vi "SaveTempData2.vi"(2 "temp data":dbl[][][](array[numeric]), 3 "Exp_params":T3={"filename"="201612011532", "ExpFilePath"=path "\\\\10.0.0.7\\takada2/DATA/HBT6/data/Test/201612011532.h5", "File Ref list"=[16777216, 33554432], "sweep_dim"=[4, 2], "sweep_list"=[], "readout_list"=["ADC0", "ADC1"], "Sweep instrument bools"=[[0, 0], [0, 0], [0, 0], [0, 0], [0, 0], [0, 0], [0, 0], [0, 0], [0, 0], [0, 0], [0, 0], [0, 0], [0, 0], [0, 0], [0, 0], [0, 0], [0, 0], [0, 0], [0, 0], [0, 0], [0, 0], [0, 0], [0, 0], [0, 0], [0, 0], [0, 0], [0, 0], [0, 0], [0, 0], [0, 0], [0, 0]], "Read out instrument bools"=[[1, 0]], "Experimental bool list"=[FALSE, TRUE], "Initial move"=[{"Name"="None", "kind"=100, "Value"=0.0}], "FPGA Ref"=refnum, "Inst_parameters"={"ConfigFilePath"=path "\\\\10.0.0.7\\takada2/DATA/HBT6/data/Configs/HBT6_ramp_1.h5", "Inst_list"=["ADC", "AWG", "Freq", "Power", "sus", "rus", "rls", "sls", "suq", "suu", "sur", "suc", "sul", "ruq", "ruu", "rur", "ruc", "rul", "rlq", "rlu", "rlr", "rlc", "rll", "slq", "slu", "slr", "slc", "sll", "tu", "t", "tl", "fast_sequence"], "fast_mode"=[1, 1], "Wait_times"=[1, 1, 1, 1], "Inst_array"=[{"Kind"=0, "Strings"=["ADC", "", "V", "ADC0;ADC1", "V;V", "1.0;1.0"], "uint64s"=[10, 2, 250000, 0, 100, 10106, 1000000, 1, 0, 1], "Doubles"=[1.0], "DAQmx take out list"=[]}, {"Kind"=7, "Strings"=["AWG", "10.0.0.4", "", "C:\\Documents and Settings\\Bauerle\\Mes documents\\Bautze\\FPGA-clean_works_1.13.6_batchtest\\Python\\AWG", "dummy", "SAWnstrig_v4.py"], "uint64s"=[2, 0, 0, 3, 0, 0, 0, 0, 0, 0, 0, 0, 0, 0], "Doubles"=[1200000000.0, 1.0, 0.0, 1.0, 0.0, 1.0, 0.0, 1.0, 0.0, 1.0, 0.0, 1.0, 0.0], "DAQmx take out list"=[]}, {"Kind"=6, "Strings"=["Freq", "0:19", "GHz"], "uint64s"=[1, 0, 0, 0, 2, 0, 0, 0], "Doubles"=[2.0, -30.0, 200.0, 100.0, 0.0, 6.000999927520752, 9.000000318337698e-06, 30.0, -145.0], "DAQmx take out list"=[]}, {"Kind"=6, "Strings"=["Power", "0:19", "GHz"], "uint64s"=[1, 0, 1, 0, 2, 0, 0, 0], "Doubles"=[2.0, -30.0, 200.0, 100.0, 0.0, 6.000999927520752, 9.000000318337698e-06, 30.0, -145.0], "DAQmx take out list"=[]}, {"Kind"=4, "Strings"=["sus", "10.0.0.2", "mV"], "uint64s"=[0, 1], "Doubles"=[1.0, -1.0, 1.0, -1.0, 1.0], "DAQmx take out list"=[]}, {"Kind"=4, "Strings"=["rus", "10.0.0.2", "mV"], "uint64s"=[0, 2], "Doubles"=[1.0, -1.0, 1.0, -1.0, 1.0], "DAQmx take out list"=[]}, {"Kind"=4, "Strings"=["rls", "10.0.0.2", "mV"], "uint64s"=[0, 3], "Doubles"=[1.0, -1.0, 1.0, -1.0, 1.0], "DAQmx take out list"=[]}, {"Kind"=4, "Strings"=["sls", "10.0.0.2", "mV"], "uint64s"=[0, 4], "Doubles"=[1.0, -1.0, 1.0, -1.0, 1.0], "DAQmx take out list"=[]}, {"Kind"=4, "Strings"=["suq", "10.0.0.2", "V"], "uint64s"=[0, 5], "Doubles"=[0.30000001192092896, -2.0, 1.0, -1.0, 1.0], "DAQmx take out list"=[]}, {"Kind"=4, "Strings"=["suu", "10.0.0.2", "V"], "uint64s"=[0, 6], "Doubles"=[0.30000001192092896, -2.0, 1.0, -1.0, 1.0], "DAQmx take out list"=[]}, {"Kind"=4, "Strings"=["sur", "10.0.0.2", "V"], "uint64s"=[0, 7], "Doubles"=[0.30000001192092896, -2.0, 1.0, -1.0, 1.0], "DAQmx take out list"=[]}, {"Kind"=4, "Strings"=["suc", "10.0.0.2", "V"], "uint64s"=[1, 0], "Doubles"=[0.30000001192092896, -2.0, 1.0, -1.0, 1.0], "DAQmx take out list"=[]}, {"Kind"=4, "Strings"=["sul", "10.0.0.2", "V"], "uint64s"=[1, 1], "Doubles"=[0.30000001192092896, -2.0, 1.0, -1.0, 1.0], "DAQmx take out list"=[]}, {"Kind"=4, "Strings"=["ruq", "10.0.0.2", "V"], "uint64s"=[1, 2], "Doubles"=[0.30000001192092896, -2.0, 1.0, -1.0, 1.0], "DAQmx take out list"=[]}, {"Kind"=4, "Strings"=["ruu", "10.0.0.2", "V"], "uint64s"=[1, 3], "Doubles"=[0.30000001192092896, -2.0, 1.0, -1.0, 1.0], "DAQmx take out list"=[]}, {"Kind"=4, "Strings"=["rur", "10.0.0.2", "V"], "uint64s"=[1, 5], "Doubles"=[0.30000001192092896, -2.0, 1.0, -1.0, 1.0], "DAQmx take out list"=[]}, {"Kind"=4, "Strings"=["ruc", "10.0.0.2", "V"], "uint64s"=[1, 6], "Doubles"=[0.30000001192092896, -2.0, 1.0, -1.0, 1.0], "DAQmx take out list"=[]}, {"Kind"=4, "Strings"=["rul", "10.0.0.2", "V"], "uint64s"=[1, 7], "Doubles"=[0.30000001192092896, -2.0, 1.0, -1.0, 1.0], "DAQmx take out list"=[]}, {"Kind"=4, "Strings"=["rlq", "10.0.0.2", "V"], "uint64s"=[2, 0], "Doubles"=[0.30000001192092896, -2.0, 1.0, -1.0, 1.0], "DAQmx take out list"=[]}, {"Kind"=4, "Strings"=["rlu", "10.0.0.2", "V"], "uint64s"=[2, 1], "Doubles"=[0.30000001192092896, -2.0, 1.0, -1.0, 1.0], "DAQmx take out list"=[]}, {"Kind"=4, "Strings"=["rlr", "10.0.0.2", "V"], "uint64s"=[2, 2], "Doubles"=[0.30000001192092896, -2.0, 1.0, -1.0, 1.0], "DAQmx take out list"=[]}, {"Kind"=4, "Strings"=["rlc", "10.0.0.2", "V"], "uint64s"=[2, 3], "Doubles"=[0.30000001192092896, -2.0, 1.0, -1.0, 1.0], "DAQmx take out list"=[]}, {"Kind"=4, "Strings"=["rll", "10.0.0.2", "V"], "uint64s"=[2, 4], "Doubles"=[0.30000001192092896, -2.0, 1.0, -1.0, 1.0], "DAQmx take out list"=[]}, {"Kind"=4, "Strings"=["slq", "10.0.0.2", "V"], "uint64s"=[2, 5], "Doubles"=[0.30000001192092896, -2.0, 1.0, -1.0, 1.0], "DAQmx take out list"=[]}, {"Kind"=4, "Strings"=["slu", "10.0.0.2", "V"], "uint64s"=[2, 6], "Doubles"=[0.30000001192092896, -2.0, 1.0, -1.0, 1.0], "DAQmx take out list"=[]}, {"Kind"=4, "Strings"=["slr", "10.0.0.2", "V"], "uint64s"=[2, 7], "Doubles"=[0.30000001192092896, -2.0, 1.0, -1.0, 1.0], "DAQmx take out list"=[]}, {"Kind"=4, "Strings"=["slc", "10.0.0.2", "V"], "uint64s"=[3, 0], "Doubles"=[0.30000001192092896, -2.0, 1.0, -1.0, 1.0], "DAQmx take out list"=[]}, {"Kind"=4, "Strings"=["sll", "10.0.0.2", "V"], "uint64s"=[3, 1], "Doubles"=[0.30000001192092896, -2.0, 1.0, -1.0, 1.0], "DAQmx take out list"=[]}, {"Kind"=4, "Strings"=["tu", "10.0.0.2", "V"], "uint64s"=[3, 2], "Doubles"=[0.30000001192092896, -2.0, 1.0, -1.0, 1.0], "DAQmx take out list"=[]}, {"Kind"=4, "Strings"=["t", "10.0.0.2", "V"], "uint64s"=[3, 3], "Doubles"=[0.30000001192092896, -2.0, 1.0, -1.0, 1.0], "DAQmx take out list"=[]}, {"Kind"=4, "Strings"=["tl", "10.0.0.2", "V"], "uint64s"=[3, 4], "Doubles"=[0.30000001192092896, -2.0, 1.0, -1.0, 1.0], "DAQmx take out list"=[]}, {"Kind"=9, "Strings"=["fast_sequence", "10.0.0.2", "V"], "uint64s"=[6661, 300, 200, 0, 0, 1, 2, 3, 4, 5, 6, 7, 16, 17, 18, 19, 20, 21, 22, 23, 0], "Doubles"=[0.5, -0.5, -1.0, -1.0], "DAQmx take out list"=[]}]}} {"File Ref list" format="%.0x"}, 4 "count":i32) -> (0 "count out":i32, 1 "Exp_params out":T3 {"File Ref list" format="%.0x"})   [LabVIEW 2010]
uses:
  <vilib>/addons/h5labview2/base/hid_t.ctl
  fpga-bitfile-ref.ctl
  <vilib>/addons/h5labview2/dataset/H5Dwrite.llb/H5Dwrite.xnode
  <vilib>/addons/h5labview2/base/lib_path.vi
  <vilib>/addons/h5labview2/base/H5Equery.vi
  <vilib>/addons/h5labview2/dataset/H5D.lvlib
  <vilib>/addons/h5labview2/space/H5S.lvlib
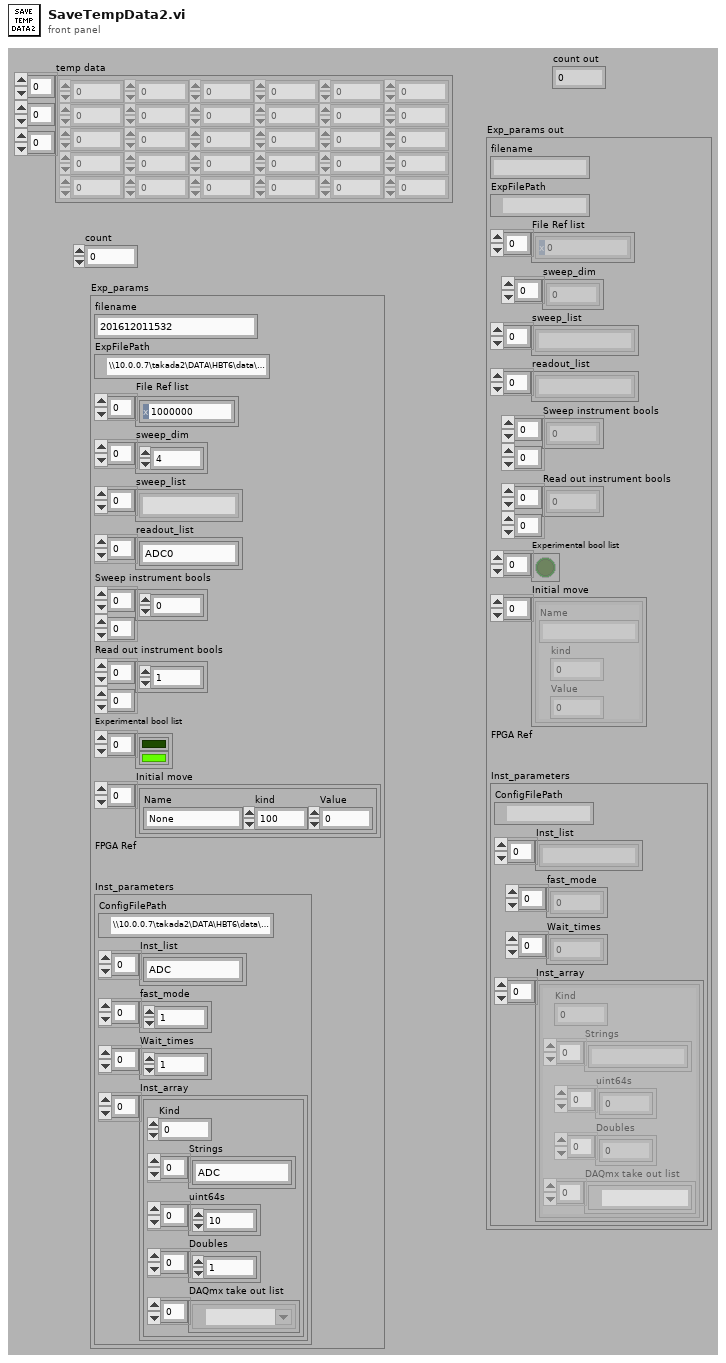
[diagram p1: front panel]
types:
  T1 = typedef "hid_t.ctl" = i32
  T2 = typedef "fpga-bitfile-ref.ctl" = refnum<k20>
  T3 = cluster{"filename":string, "ExpFilePath":path, "File Ref list":T1[], "sweep_dim":u64[], "sweep_list":string[], "readout_list":string[], "Sweep instrument bools":u64[][], "Read out instrument bools":u64[][], "Experimental bool list":bool[], "Initial move":cluster{"Name":string, "kind":u64, "Value":dbl}[], "FPGA Ref":T2, "Inst_parameters":cluster{"ConfigFilePath":path, "Inst_list":string[], "fast_mode":u8[], "Wait_times":u64[], "Inst_array":cluster{"Kind":u16, "Strings":string[], "uint64s":u64[], "Doubles":dbl[], "DAQmx take out list":refnum<k21>[]}[]}}
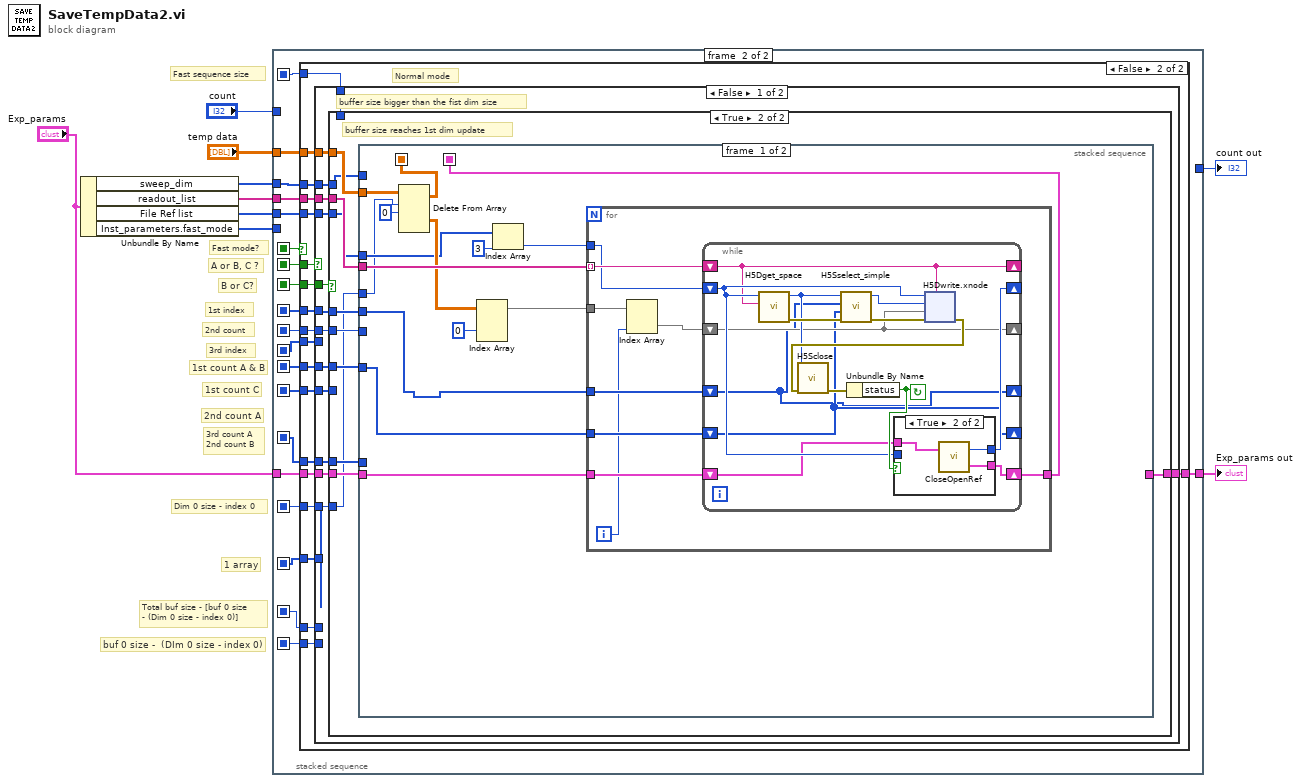
[diagram p0: block diagram]
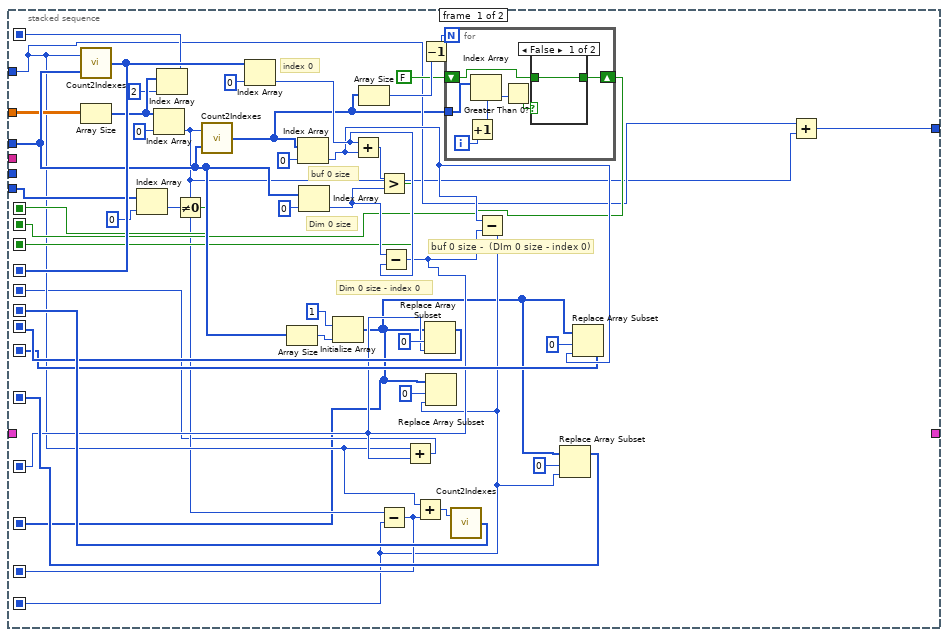
[diagram p2: hidden frame]
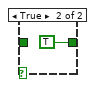
[diagram p3: hidden frame]
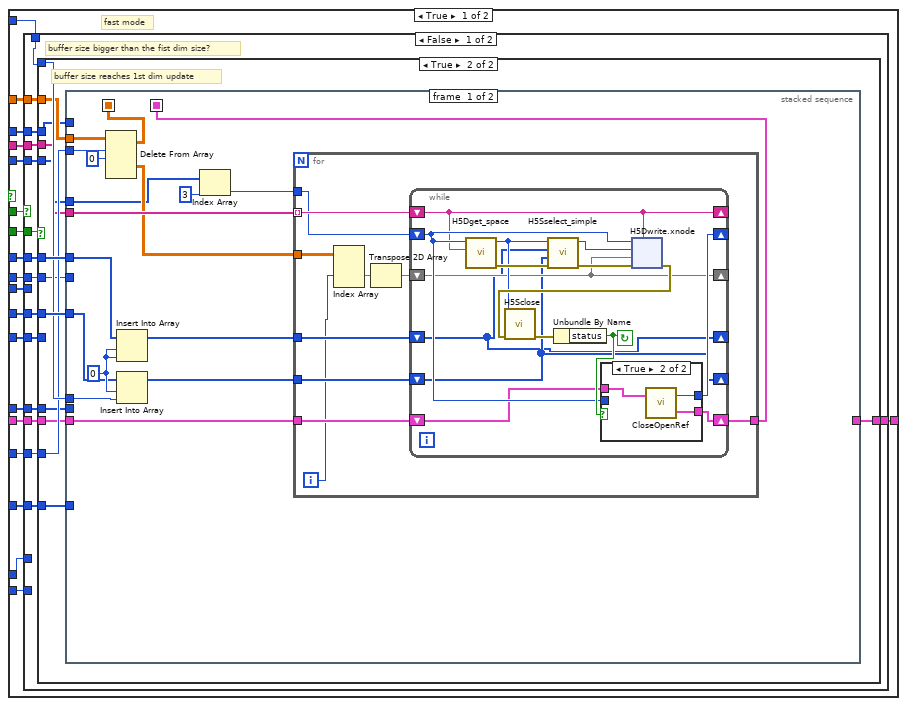
[diagram p4: hidden frame]
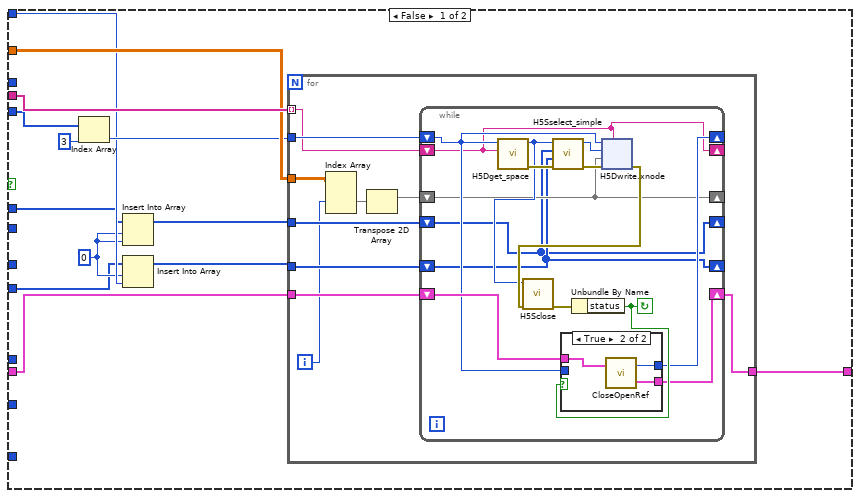
[diagram p5: hidden frame]
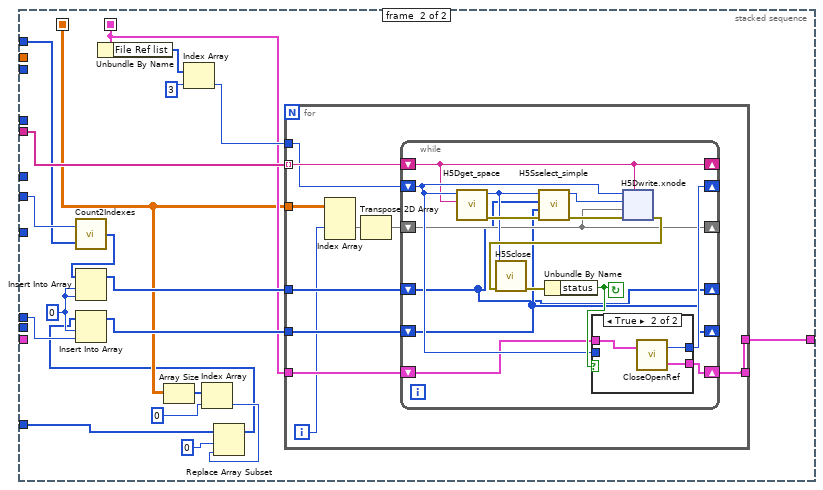
[diagram p8: hidden frame]
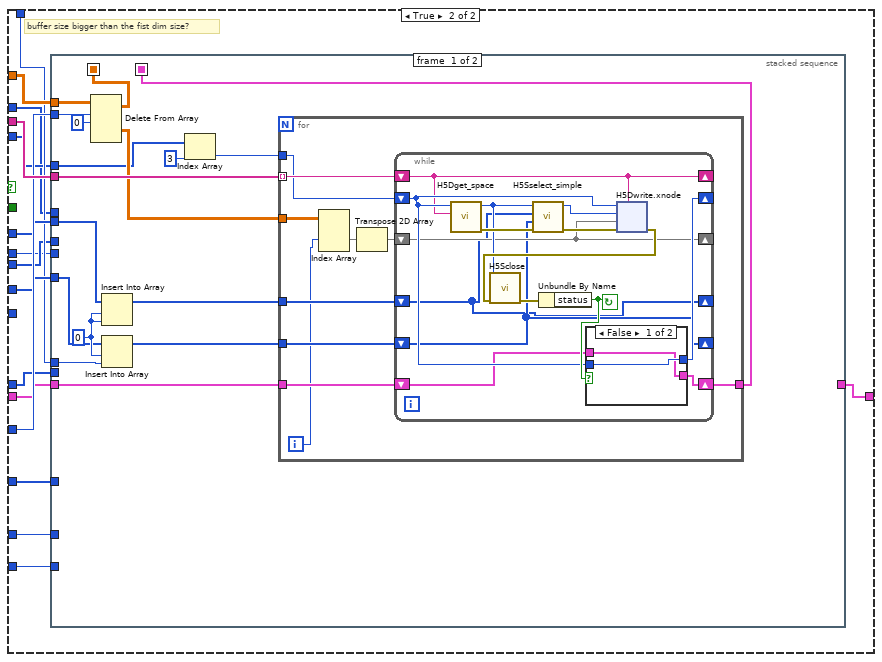
[diagram p10: hidden frame]
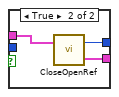
[diagram p11: hidden frame]
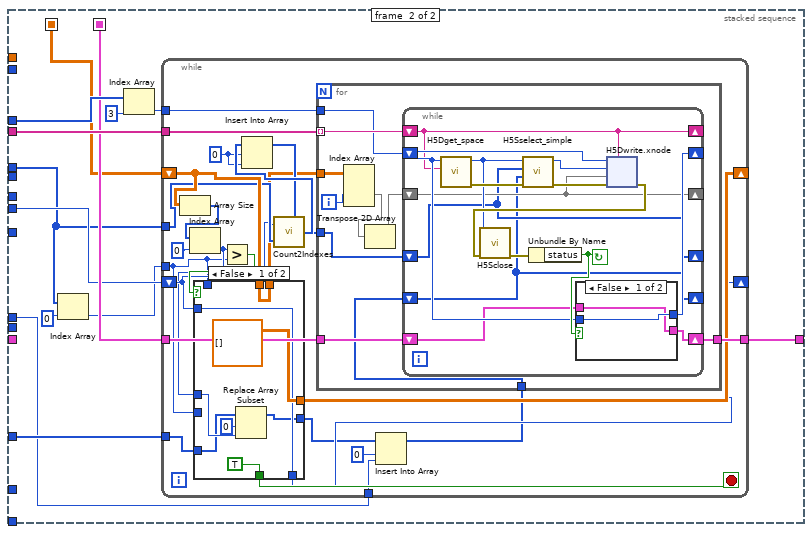
[diagram p12: hidden frame]
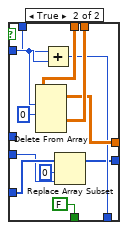
[diagram p13: hidden frame]
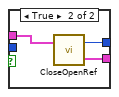
[diagram p14: hidden frame]
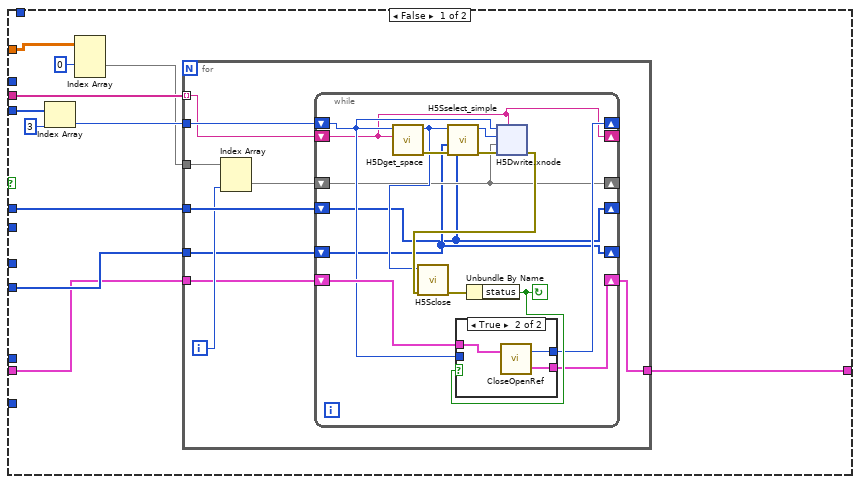
[diagram p15: hidden frame]
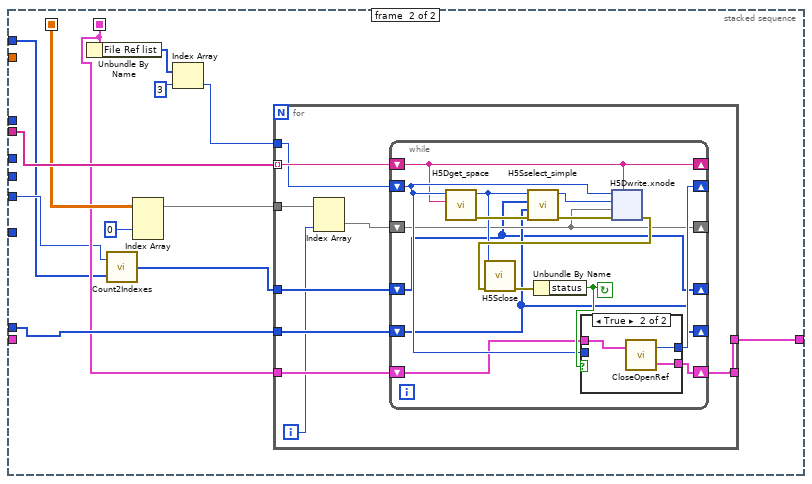
[diagram p18: hidden frame]
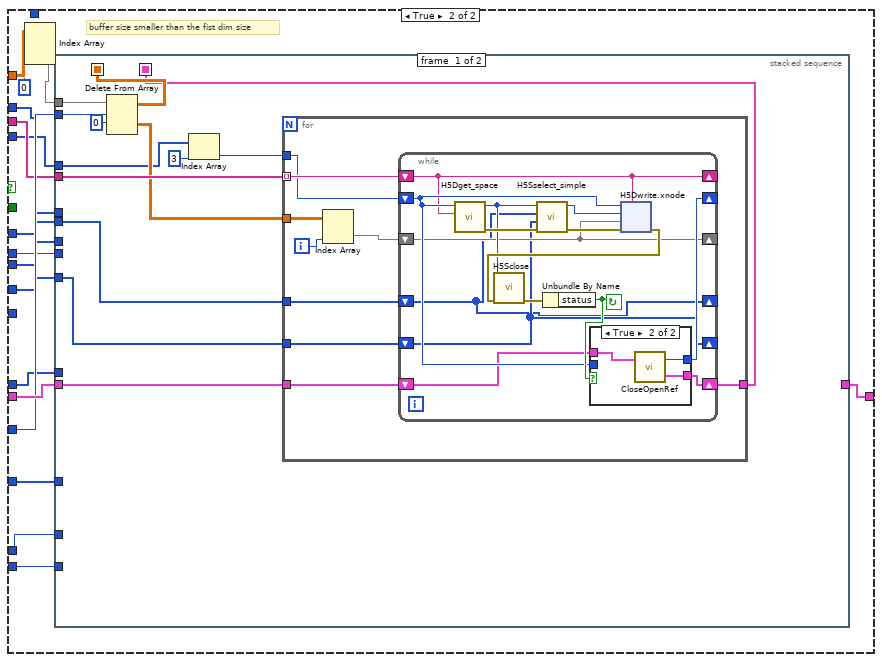
[diagram p20: hidden frame]
diagram:
  # "1 array"
  # "buf 0 size -  (DIm 0 size - index 0)"
  # "Total buf size - [buf 0 size\n- (Dim 0 size - index 0)]"
  # "Dim 0 size - index 0"
  # "Fast sequence size"
  # "B or C?"
  # "A or B, C ?"
  # "Fast mode?"
  # "3rd count A\n2nd count B"
  # "2nd count A"
  # "1st count C"
  # "1st count A & B"
  # "3rd index"
  # "2nd count"
  # "1st index"
  n1 = Unbundle By Name("Exp_params") -> ("sweep_dim"=w6:u64[], "readout_list"=w5:string[], "File Ref list"=w7:T1[], "Inst_parameters.fast_mode"=w4:u8[])
  n2 = stacked-sequence {
    seq-local: [w48 _] -> [_ w75]
    seq-local: [w11 _] -> [_ w67]
    seq-local: [w36 _] -> [_ w66]
    seq-local: [w35 _] -> [_ w71]
    seq-local: [w32 _] -> [_ w74]
    seq-local: [w29 _] -> [_ w68]
    seq-local: [w22 _] -> [_ w81]
    seq-local: [w26 _] -> [_ w80]
    seq-local: [w27 _] -> [_ w79]
    seq-local: [w19 _] -> [_ w72]
    seq-local: [w18 _] -> [_ w70]
    seq-local: [w14 _] -> [_ w65]
    seq-local: [w13 _] -> [_ w64]
    seq-local: [w10 _] -> [_ w62]
    tunnel: "count" -> [w17 _]
    tunnel: "temp data" -> [w28 w78]
    tunnel: w7 -> [_ w76]
    tunnel: w6 -> [w38 w63]
    tunnel: w5 -> [_ w77]
    tunnel: w4 -> [w25 _]
    tunnel: "Exp_params" -> [_ w73]
    tunnel: [_ w69] -> w1
    tunnel: [w16 _] -> w2
    frame #0 {
      # "buf 0 size -  (DIm 0 size - index 0)"
      # "Dim 0 size - index 0"
      # "Dim 0 size"
      # "buf 0 size"
      # "index 0"
      n3 = call "Count2Indexes.vi"("sweep_dim"=w38, "Count"=w17) -> ("Indexes"=w48:u64[])
      n4 = Array Size(array=w28) -> (size(s)=w21:i32[])
      n5 = Index Array(array=w25, index=0) -> (element=w23:u8)
      n6 = Index Array(array=w21, index=0) -> (element=w15:i32)
      n7 = Index Array(array=w21, index=2) -> (element=w19:i32)
      n8 = Not Equal To 0?(x=w23) -> (x != 0?=w22:bool)
      n9 = call "Count2Indexes.vi"("sweep_dim"=w38, "Count"=w15) -> ("Indexes"=w12:u64[])
      n10 = Index Array(array=w48, index=0) -> (element=w43:u64)
      n11 = Array Size(array=w38) -> (size(s)=w42:i32)
      n12 = Index Array(array=w12, index=0) -> (element=w33:u64)
      n13 = Index Array(array=w38, index=0) -> (element=w31:u64)
      n14 = Initialize Array(1, w42) -> (w10:i32[])
      n15 = Add(x=w43, y=w33) -> (x+y=w47:u64)
      n16 = Array Size(array=w12) -> (size(s)=w46:i32)
      n17 = Greater?(x=w47, y=w31) -> (0:w27:bool)
      n18 = Subtract(x=w31, y=w43) -> (x-y=w18:u64)
      n19 = Add(x=w17, y=w18) -> (x+y=w11:u64)
      n20 = Decrement(x=w46) -> (x-1=w45:i32)
      n21 = Replace Array Subset(array=w10, new element=w18, index=0) -> (w35:i32[])
      n22 = for {
        N: w45 -> [_]
        tunnel: w12 -> [w59]
        shift-right: [w53] -> w26
        shift-left: FALSE -> [w54]
        i -> [w58]
        n23 = Increment(x=w58) -> (x+1=w57:i32)
        n24 = Index Array(array=w59, index=w57) -> (element=w56:u64)
        n25 = Greater Than 0?(x=w56) -> (x > 0?=w55:bool)
        n26 = case shown="False" w55 {
          tunnel: w54 -> [w60 _]
          tunnel: [w60 TRUE] -> w53
          frame False {
          }
          frame True {
          }
        }
      }
      n27 = Subtract(x=w33, y=w18) -> (x-y=w13:u64)
      n28 = Subtract(x=w15, y=w13) -> (x-y=w14:u64)
      n29 = Add(x=w17, y=w14) -> (x+y=w37:u64)
      n30 = Replace Array Subset(array=w10, new element=w13, index=0) -> ()  [unwired: 1 out]
      n31 = call "Count2Indexes.vi"("Count"=w37) -> ("Indexes"=w36:u64[])  [unwired: 1 in]
      n32 = Replace Array Subset(array=w10, new element=w13, index=0) -> (w29:i32[])
      n33 = Replace Array Subset(array=w10, new element=w33, index=0) -> (w32:i32[])
      n34 = Add(x=w17, y=w15) -> (x+y=w16:i32)
    }
    frame #1 {
      n35 = case shown="False" w81 {
        tunnel: w80 -> [w100 w527]
        tunnel: w79 -> [w99 w526]
        tunnel: w78 -> [w97 w525]
        tunnel: w77 -> [w98 w524]
        tunnel: w76 -> [w96 w523]
        tunnel: w75 -> [w93 w522]
        tunnel: w74 -> [w92 w521]
        tunnel: w73 -> [w95 w520]
        tunnel: w72 -> [w94 w517]
        tunnel: w71 -> [w91 w518]
        tunnel: w70 -> [w90 w514]
        tunnel: [w89 w519] -> w69
        tunnel: w68 -> [w88 w516]
        tunnel: w67 -> [w87 w515]
        tunnel: w66 -> [w86 w509]
        tunnel: w65 -> [w85 w513]
        tunnel: w64 -> [w84 w512]
        tunnel: w63 -> [w83 w511]
        tunnel: w62 -> [w82 w510]
        frame True {
          # "fast mode"
          n36 = case shown="False" w100 {
            tunnel: w99 -> [w115 _]
            tunnel: w98 -> [w114 w337]
            tunnel: w97 -> [w113 w338]
            tunnel: w96 -> [w112 w329]
            tunnel: w95 -> [w111 w332]
            tunnel: w94 -> [w110 w333]
            tunnel: w93 -> [w109 w335]
            tunnel: w92 -> [w108 _]
            tunnel: w91 -> [w107 w334]
            tunnel: w90 -> [w106 w336]
            tunnel: [w105 w327] -> w89
            tunnel: w88 -> [w104 w330]
            tunnel: w87 -> [w103 w328]
            tunnel: w86 -> [_ w331]
            tunnel: w85 -> [_ w326]
            tunnel: w84 -> [_ w325]
            tunnel: w83 -> [w102 w324]
            tunnel: w82 -> [w101 w323]
            frame False {
              # "buffer size bigger than the fist dim size?"
              n37 = case shown="True" w115 {
                tunnel: w114 -> [w128 w184]
                tunnel: w113 -> [w127 w186]
                tunnel: w112 -> [w125 w183]
                tunnel: w111 -> [w123 w182]
                tunnel: w110 -> [w122 w187]
                tunnel: w109 -> [w120 w188]
                tunnel: w108 -> [w119 _]
                tunnel: w107 -> [_ w189]
                tunnel: w106 -> [_ w185]
                tunnel: [w116 w179] -> w105
                tunnel: w104 -> [_ w181]
                tunnel: w103 -> [_ w180]
                tunnel: w102 -> [_ w178]
                tunnel: w101 -> [_ w177]
                frame False {
                  w121 = 0
                  n38 = Index Array(array=w125, index=3) -> (element=w124:T1)
                  n39 = Insert Into Array(array=w120, index=w121, new element=w121) -> (w118:u64[])
                  n40 = Insert Into Array(array=w119, index=w121, new element=w122) -> (w117:i32[])
                  n41 = for {
                    tunnel: w118 -> [w138]
                    tunnel: w124 -> [w137]
                    tunnel: w128 -> [w136] mode=indexing
                    tunnel: w127 -> [w135]
                    tunnel: w117 -> [w133]
                    tunnel: w123 -> [w132]
                    tunnel: [w131] -> w116
                    i -> [w130]
                    n42 = Index Array(array=w135, index (dim 1)=w130) -> (element=w134:dbl[][])  [unwired: 2 in]
                    n43 = Transpose 2D Array(2D array=w134) -> (transposed array=w129:dbl[][])
                    n44 = while {
                      shift-right: [w139] -> _
                      shift-left: w138 -> [w139]
                      shift-right: [w144] -> _
                      shift-left: w137 -> [w145]
                      shift-right: [w143] -> _
                      shift-left: w129 -> [w143]
                      shift-right: [w140] -> _
                      shift-left: w133 -> [w140]
                      shift-right: [w141] -> w131
                      shift-left: w132 -> [w146]
                      shift-right: [w142] -> _
                      shift-left: w136 -> [w142]
                      stop <- w147 continue-if-true
                      n45 = call <vilib>:"H5Dget_space.vi"("obj (.)"=w142, "ref in"=w145) -> ("error out"=w153:errorcluster, "space out"=w148:T1)  [unwired: 8 in]
                      n46 = call <vilib>:"H5Sselect_simple.vi"("error in (no error)"=w153, "count"=w140, "start"=w139, "space in"=w148) -> ("error out"=w152:errorcluster, "space out"=w151:T1)  [unwired: 6 in]
                      n47 = xnode "H5Dwrite.xnode"("dataset name"=w142, "error in (no error)"=w152, "data"=w143, "file space"=w151, "ref in"=w145) -> ("error out"=w149:errorcluster)  [unwired: 2 in, 2 out]
                      n48 = call <vilib>:"H5Sclose.vi"("error in (no error)"=w149, "space in"=w148) -> ("error out"=w150:errorcluster)  [unwired: 9 in]
                      n49 = Unbundle By Name(w150) -> ("status"=w147:bool)
                      n50 = case shown="True" w147 {
                        tunnel: w145 -> [w155 _]
                        tunnel: [w155 w157] -> w144
                        tunnel: w146 -> [w154 w158]
                        tunnel: [w154 w156] -> w141
                        frame False {
                        }
                        frame True {
                          n51 = call "CloseOpenRef.vi"("Exp_params"=w158) -> ("Exp_params_out"=w156:T3, "group out"=w157:T1)  [unwired: 1 in]
                        }
                      }
                    }
                  }
                }
                frame True {
                  # "buffer size reaches 1st dim update"
                  n52 = stacked-sequence {
                    seq-local: [w199 _] -> [_ w261]
                    seq-local: [w190 _] -> [_ w265]
                    tunnel: w189 -> [w205 _]
                    tunnel: w188 -> [w204 _]
                    tunnel: w187 -> [w203 w269]
                    tunnel: w186 -> [w202 _]
                    tunnel: w185 -> [w201 _]
                    tunnel: w184 -> [w198 w274]
                    tunnel: w183 -> [w195 _]
                    tunnel: w182 -> [w191 _]
                    tunnel: w181 -> [_ _]
                    tunnel: w180 -> [_ w264]
                    tunnel: [_ w266] -> w179
                    tunnel: w178 -> [_ w262]
                    tunnel: w177 -> [_ w258]
                    frame #0 {
                      w206 = 0
                      n53 = Delete From Array(array=w202, length=w201, index (dim 0)=0) -> (deleted portion=w197:dbl[][][], array with subset deleted=w199:dbl[][][])  [unwired: 2 in]
                      n54 = Insert Into Array(array=w204, index=w206, new element=w206) -> (w192:u64[])
                      n55 = Insert Into Array(array=w205, index=w206, new element=w203) -> (w193:i32[])
                      n56 = Index Array(array=w195, index=3) -> (element=w194:T1)
                      n57 = for {
                        tunnel: w198 -> [w214] mode=indexing
                        tunnel: w197 -> [w216]
                        tunnel: w194 -> [w213]
                        tunnel: w193 -> [w212]
                        tunnel: w192 -> [w211]
                        tunnel: w191 -> [w210]
                        tunnel: [w209] -> w190
                        i -> [w208]
                        n58 = Index Array(array=w216, index (dim 1)=w208) -> (element=w215:dbl[][])  [unwired: 2 in]
                        n59 = Transpose 2D Array(2D array=w215) -> (transposed array=w207:dbl[][])
                        n60 = while {
                          shift-right: [w222] -> _
                          shift-left: w207 -> [w222]
                          shift-right: [w217] -> _
                          shift-left: w214 -> [w217]
                          shift-right: [w223] -> _
                          shift-left: w213 -> [w224]
                          shift-right: [w220] -> w209
                          shift-left: w210 -> [w221]
                          shift-right: [w219] -> _
                          shift-left: w212 -> [w219]
                          shift-right: [w218] -> _
                          shift-left: w211 -> [w218]
                          stop <- w225 continue-if-true
                          n61 = call <vilib>:"H5Dget_space.vi"("obj (.)"=w217, "ref in"=w224) -> ("error out"=w231:errorcluster, "space out"=w226:T1)  [unwired: 8 in]
                          n62 = call <vilib>:"H5Sselect_simple.vi"("error in (no error)"=w231, "count"=w219, "start"=w218, "space in"=w226) -> ("error out"=w230:errorcluster, "space out"=w229:T1)  [unwired: 6 in]
                          n63 = xnode "H5Dwrite.xnode"("dataset name"=w217, "error in (no error)"=w230, "data"=w222, "file space"=w229, "ref in"=w224) -> ("error out"=w227:errorcluster)  [unwired: 2 in, 2 out]
                          n64 = call <vilib>:"H5Sclose.vi"("error in (no error)"=w227, "space in"=w226) -> ("error out"=w228:errorcluster)  [unwired: 9 in]
                          n65 = Unbundle By Name(w228) -> ("status"=w225:bool)
                          n66 = case shown="True" w225 {
                            tunnel: w224 -> [w233 _]
                            tunnel: [w233 w235] -> w223
                            tunnel: w221 -> [w232 w236]
                            tunnel: [w232 w234] -> w220
                            frame False {
                            }
                            frame True {
                              n67 = call "CloseOpenRef.vi"("Exp_params"=w236) -> ("Exp_params_out"=w234:T3, "group out"=w235:T1)  [unwired: 1 in]
                            }
                          }
                        }
                      }
                    }
                    frame #1 {
                      w270 = 0
                      n68 = call "Count2Indexes.vi"("sweep_dim"=w262, "Count"=w264) -> ("Indexes"=w263:u64[])
                      n69 = Insert Into Array(array=w263, index=w270, new element=w270) -> (w267:u64[])
                      n70 = Unbundle By Name(w265) -> ("File Ref list"=w273:T1[])
                      n71 = Array Size(array=w261) -> (size(s)=w260:i32[])
                      n72 = Index Array(array=w273, index=3) -> (element=w271:T1)
                      n73 = Index Array(array=w260, index=0) -> (element=w257:i32)
                      n74 = Replace Array Subset(array=w258, new element=w257, index=0) -> (w255:i32[])
                      n75 = Insert Into Array(array=w255, index=w270, new element=w269) -> (w268:i32[])
                      n76 = for {
                        tunnel: w274 -> [w282] mode=indexing
                        tunnel: w261 -> [w284]
                        tunnel: w271 -> [w281]
                        tunnel: w268 -> [w280]
                        tunnel: w267 -> [w279]
                        tunnel: w265 -> [w278]
                        tunnel: [w277] -> _
                        tunnel: [w277] -> w266
                        i -> [w276]
                        n77 = Index Array(array=w284, index (dim 1)=w276) -> (element=w283:dbl[][])  [unwired: 2 in]
                        n78 = Transpose 2D Array(2D array=w283) -> (transposed array=w275:dbl[][])
                        n79 = while {
                          shift-right: [w290] -> _
                          shift-left: w275 -> [w290]
                          shift-right: [w285] -> _
                          shift-left: w282 -> [w285]
                          shift-right: [w291] -> _
                          shift-left: w281 -> [w292]
                          shift-right: [w288] -> w277
                          shift-left: w278 -> [w289]
                          shift-right: [w287] -> _
                          shift-left: w280 -> [w287]
                          shift-right: [w286] -> _
                          shift-left: w279 -> [w286]
                          stop <- w293 continue-if-true
                          n80 = call <vilib>:"H5Dget_space.vi"("obj (.)"=w285, "ref in"=w292) -> ("error out"=w299:errorcluster, "space out"=w294:T1)  [unwired: 8 in]
                          n81 = call <vilib>:"H5Sselect_simple.vi"("error in (no error)"=w299, "count"=w287, "start"=w286, "space in"=w294) -> ("error out"=w298:errorcluster, "space out"=w297:T1)  [unwired: 6 in]
                          n82 = xnode "H5Dwrite.xnode"("dataset name"=w285, "error in (no error)"=w298, "data"=w290, "file space"=w297, "ref in"=w292) -> ("error out"=w295:errorcluster)  [unwired: 2 in, 2 out]
                          n83 = call <vilib>:"H5Sclose.vi"("error in (no error)"=w295, "space in"=w294) -> ("error out"=w296:errorcluster)  [unwired: 9 in]
                          n84 = Unbundle By Name(w296) -> ("status"=w293:bool)
                          n85 = case shown="True" w293 {
                            tunnel: w292 -> [w301 _]
                            tunnel: [w301 w303] -> w291
                            tunnel: w289 -> [w300 w304]
                            tunnel: [w300 w302] -> w288
                            frame False {
                            }
                            frame True {
                              n86 = call "CloseOpenRef.vi"("Exp_params"=w304) -> ("Exp_params_out"=w302:T3, "group out"=w303:T1)  [unwired: 1 in]
                            }
                          }
                        }
                      }
                    }
                  }
                }
              }
            }
            frame True {
              # "buffer size bigger than the fist dim size?"
              n87 = stacked-sequence {
                seq-local: [w348 _] -> [_ w405]
                seq-local: [w340 _] -> [_ w412]
                tunnel: w334 -> [w354 _]
                tunnel: w335 -> [w353 _]
                tunnel: w333 -> [w352 w406]
                tunnel: w338 -> [w351 _]
                tunnel: w336 -> [w350 _]
                tunnel: w337 -> [w347 w416]
                tunnel: w329 -> [w344 w414]
                tunnel: w332 -> [w341 _]
                tunnel: w330 -> [_ _]
                tunnel: w331 -> [_ _]
                tunnel: [_ w404] -> w327
                tunnel: w328 -> [_ w411]
                tunnel: w326 -> [_ _]
                tunnel: w325 -> [_ _]
                tunnel: w324 -> [_ w410]
                tunnel: w323 -> [_ w407]
                frame #0 {
                  w355 = 0
                  n88 = Delete From Array(array=w351, length=w350, index (dim 0)=0) -> (deleted portion=w346:dbl[][][], array with subset deleted=w348:dbl[][][])  [unwired: 2 in]
                  n89 = Insert Into Array(array=w353, index=w355, new element=w355) -> (w342:u64[])
                  n90 = Insert Into Array(array=w354, index=w355, new element=w352) -> (w339:i32[])
                  n91 = Index Array(array=w344, index=3) -> (element=w343:T1)
                  n92 = for {
                    tunnel: w347 -> [w363] mode=indexing
                    tunnel: w346 -> [w365]
                    tunnel: w343 -> [w362]
                    tunnel: w339 -> [w361]
                    tunnel: w342 -> [w360]
                    tunnel: w341 -> [w359]
                    tunnel: [w358] -> w340
                    i -> [w357]
                    n93 = Index Array(array=w365, index (dim 1)=w357) -> (element=w364:dbl[][])  [unwired: 2 in]
                    n94 = Transpose 2D Array(2D array=w364) -> (transposed array=w356:dbl[][])
                    n95 = while {
                      shift-right: [w371] -> _
                      shift-left: w356 -> [w371]
                      shift-right: [w366] -> _
                      shift-left: w363 -> [w366]
                      shift-right: [w372] -> _
                      shift-left: w362 -> [w373]
                      shift-right: [w369] -> w358
                      shift-left: w359 -> [w370]
                      shift-right: [w368] -> _
                      shift-left: w361 -> [w368]
                      shift-right: [w367] -> _
                      shift-left: w360 -> [w367]
                      stop <- w374 continue-if-true
                      n96 = call <vilib>:"H5Dget_space.vi"("obj (.)"=w366, "ref in"=w373) -> ("error out"=w380:errorcluster, "space out"=w375:T1)  [unwired: 8 in]
                      n97 = call <vilib>:"H5Sselect_simple.vi"("error in (no error)"=w380, "count"=w368, "start"=w367, "space in"=w375) -> ("error out"=w379:errorcluster, "space out"=w378:T1)  [unwired: 6 in]
                      n98 = xnode "H5Dwrite.xnode"("dataset name"=w366, "error in (no error)"=w379, "data"=w371, "file space"=w378, "ref in"=w373) -> ("error out"=w376:errorcluster)  [unwired: 2 in, 2 out]
                      n99 = call <vilib>:"H5Sclose.vi"("error in (no error)"=w376, "space in"=w375) -> ("error out"=w377:errorcluster)  [unwired: 9 in]
                      n100 = Unbundle By Name(w377) -> ("status"=w374:bool)
                      n101 = case shown="False" w374 {
                        tunnel: w373 -> [w382 _]
                        tunnel: [w382 w384] -> w372
                        tunnel: w370 -> [w381 w385]
                        tunnel: [w381 w383] -> w369
                        frame False {
                        }
                        frame True {
                          n102 = call "CloseOpenRef.vi"("Exp_params"=w385) -> ("Exp_params_out"=w383:T3, "group out"=w384:T1)  [unwired: 1 in]
                        }
                      }
                    }
                  }
                }
                frame #1 {
                  n103 = Index Array(array=w410, index=0) -> (element=w408:u64)
                  n104 = Index Array(array=w414, index=3) -> (element=w413:T1)
                  n105 = while {
                    tunnel: w416 -> [w440]
                    tunnel: w413 -> [w439]
                    tunnel: w412 -> [w438]
                    tunnel: [w437] -> w404
                    shift-right: [w431] -> _
                    shift-left: w405 -> [w433]
                    tunnel: w410 -> [w429]
                    shift-right: [w430] -> _
                    shift-left: w411 -> [w428]
                    tunnel: w408 -> [w422]
                    tunnel: w407 -> [w421]
                    tunnel: w406 -> [w418]
                    stop <- w432 stop-if-true
                    w426 = 0
                    n106 = Array Size(array=w433) -> (size(s)=w436:i32[])
                    n107 = Index Array(array=w436, index=0) -> (element=w423:i32)
                    n108 = Greater?(x=w423, y=w422) -> (0:w434:bool)
                    n109 = case shown="False" w434 {
                      tunnel: w428 -> [w445 w460]
                      tunnel: w422 -> [_ w456]
                      tunnel: w433 -> [w447 w459]
                      tunnel: [w447 w458] -> w424
                      tunnel: [TRUE FALSE] -> w432
                      tunnel: [dbl[][][] [] w454] -> w431
                      tunnel: [w445 w453] -> w430
                      tunnel: w423 -> [w442 _]
                      tunnel: w422 -> [_ w451]
                      tunnel: w421 -> [w441 w452]
                      tunnel: [w443 w449] -> w420
                      frame False {
                        n110 = Replace Array Subset(array=w441, new element=w442, index=0) -> (w443:i32[])
                      }
                      frame True {
                        n111 = Delete From Array(array=w459, length=w456, index (dim 0)=0) -> (deleted portion=w458:dbl[][][], array with subset deleted=w454:dbl[][][])  [unwired: 2 in]
                        n112 = Add(x=w456, y=w460) -> (x+y=w453:u64)
                        n113 = Replace Array Subset(array=w452, new element=w451, index=0) -> (w449:i32[])
                      }
                    }
                    n114 = call "Count2Indexes.vi"("sweep_dim"=w429, "Count"=w428) -> ("Indexes"=w427:u64[])
                    n115 = Insert Into Array(array=w427, index=w426, new element=w426) -> (w425:u64[])
                    n116 = Insert Into Array(array=w420, index=0, new element=w418) -> (w417:i32[])
                    n117 = for {
                      tunnel: w440 -> [w469] mode=indexing
                      tunnel: w424 -> [w470]
                      tunnel: w439 -> [w468]
                      tunnel: w438 -> [w467]
                      tunnel: [w466] -> w437
                      tunnel: w425 -> [w465]
                      tunnel: w417 -> [w464]
                      i -> [w463]
                      n118 = Index Array(array=w470, index (dim 1)=w463) -> (element=w462:dbl[][])  [unwired: 2 in]
                      n119 = Transpose 2D Array(2D array=w462) -> (transposed array=w461:dbl[][])
                      n120 = while {
                        shift-right: [w476] -> _
                        shift-left: w461 -> [w476]
                        shift-right: [w473] -> _
                        shift-left: w469 -> [w473]
                        shift-right: [w477] -> _
                        shift-left: w468 -> [w478]
                        shift-right: [w474] -> w466
                        shift-left: w467 -> [w475]
                        shift-right: [w471] -> _
                        shift-left: w464 -> [w471]
                        shift-right: [w472] -> _
                        shift-left: w465 -> [w472]
                        stop <- w479 continue-if-true
                        n121 = call <vilib>:"H5Dget_space.vi"("obj (.)"=w473, "ref in"=w478) -> ("error out"=w485:errorcluster, "space out"=w480:T1)  [unwired: 8 in]
                        n122 = call <vilib>:"H5Sselect_simple.vi"("error in (no error)"=w485, "count"=w471, "start"=w472, "space in"=w480) -> ("error out"=w484:errorcluster, "space out"=w483:T1)  [unwired: 6 in]
                        n123 = xnode "H5Dwrite.xnode"("dataset name"=w473, "error in (no error)"=w484, "data"=w476, "file space"=w483, "ref in"=w478) -> ("error out"=w481:errorcluster)  [unwired: 2 in, 2 out]
                        n124 = call <vilib>:"H5Sclose.vi"("error in (no error)"=w481, "space in"=w480) -> ("error out"=w482:errorcluster)  [unwired: 9 in]
                        n125 = Unbundle By Name(w482) -> ("status"=w479:bool)
                        n126 = case shown="False" w479 {
                          tunnel: w478 -> [w487 _]
                          tunnel: [w487 w489] -> w477
                          tunnel: w475 -> [w486 w490]
                          tunnel: [w486 w488] -> w474
                          frame False {
                          }
                          frame True {
                            n127 = call "CloseOpenRef.vi"("Exp_params"=w490) -> ("Exp_params_out"=w488:T3, "group out"=w489:T1)  [unwired: 1 in]
                          }
                        }
                      }
                    }
                  }
                }
              }
            }
          }
        }
        frame False {
          # "Normal mode"
          n128 = case shown="False" w527 {
            tunnel: w526 -> [w541 _]
            tunnel: w525 -> [w540 w735]
            tunnel: w524 -> [w539 w746]
            tunnel: w523 -> [w538 w745]
            tunnel: w522 -> [w537 w744]
            tunnel: w521 -> [w536 _]
            tunnel: w520 -> [w535 w748]
            tunnel: [w534 w749] -> w519
            tunnel: w518 -> [w533 w743]
            tunnel: w517 -> [w532 _]
            tunnel: w516 -> [w531 w736]
            tunnel: w515 -> [w530 w739]
            tunnel: w514 -> [w529 w747]
            tunnel: w513 -> [_ w742]
            tunnel: w512 -> [_ w741]
            tunnel: w511 -> [w528 w740]
            tunnel: w510 -> [_ w738]
            tunnel: w509 -> [_ w737]
            frame False {
              # "buffer size bigger than the fist dim size"
              n129 = case shown="True" w541 {
                tunnel: w540 -> [w547 w609]
                tunnel: w539 -> [w548 w608]
                tunnel: w538 -> [w552 w607]
                tunnel: w537 -> [w550 w606]
                tunnel: w536 -> [w544 _]
                tunnel: w535 -> [w543 w604]
                tunnel: [w542 w610] -> w534
                tunnel: w533 -> [_ w605]
                tunnel: w532 -> [_ _]
                tunnel: w531 -> [_ w603]
                tunnel: w530 -> [_ w602]
                tunnel: w529 -> [_ w601]
                tunnel: w528 -> [_ w600]
                frame False {
                  n130 = Index Array(array=w552, index=3) -> (element=w549:T1)
                  n131 = Index Array(array=w547, index (dim 1)=0) -> (element=w545:dbl[][])  [unwired: 2 in]
                  n132 = for {
                    tunnel: w550 -> [w561]
                    tunnel: w549 -> [w560]
                    tunnel: w548 -> [w559] mode=indexing
                    tunnel: w545 -> [w558]
                    tunnel: w544 -> [w555]
                    tunnel: w543 -> [w554]
                    tunnel: [w553] -> w542
                    i -> [w557]
                    n133 = Index Array(array=w558, index (col)=w557) -> (element=w556:dbl[])  [unwired: 1 in]
                    n134 = while {
                      shift-right: [w562] -> _
                      shift-left: w561 -> [w562]
                      shift-right: [w567] -> _
                      shift-left: w560 -> [w568]
                      shift-right: [w566] -> _
                      shift-left: w556 -> [w566]
                      shift-right: [w563] -> _
                      shift-left: w555 -> [w563]
                      shift-right: [w564] -> w553
                      shift-left: w554 -> [w569]
                      shift-right: [w565] -> _
                      shift-left: w559 -> [w565]
                      stop <- w570 continue-if-true
                      n135 = call <vilib>:"H5Dget_space.vi"("obj (.)"=w565, "ref in"=w568) -> ("error out"=w576:errorcluster, "space out"=w571:T1)  [unwired: 8 in]
                      n136 = call <vilib>:"H5Sselect_simple.vi"("error in (no error)"=w576, "count"=w563, "start"=w562, "space in"=w571) -> ("error out"=w575:errorcluster, "space out"=w574:T1)  [unwired: 6 in]
                      n137 = xnode "H5Dwrite.xnode"("dataset name"=w565, "error in (no error)"=w575, "data"=w566, "file space"=w574, "ref in"=w568) -> ("error out"=w572:errorcluster)  [unwired: 2 in, 2 out]
                      n138 = call <vilib>:"H5Sclose.vi"("error in (no error)"=w572, "space in"=w571) -> ("error out"=w573:errorcluster)  [unwired: 9 in]
                      n139 = Unbundle By Name(w573) -> ("status"=w570:bool)
                      n140 = case shown="True" w570 {
                        tunnel: w568 -> [w578 _]
                        tunnel: [w578 w580] -> w567
                        tunnel: w569 -> [w577 w581]
                        tunnel: [w577 w579] -> w564
                        frame False {
                        }
                        frame True {
                          n141 = call "CloseOpenRef.vi"("Exp_params"=w581) -> ("Exp_params_out"=w579:T3, "group out"=w580:T1)  [unwired: 1 in]
                        }
                      }
                    }
                  }
                }
                frame True {
                  # "buffer size reaches 1st dim update"
                  n142 = stacked-sequence {
                    seq-local: [w623 _] -> [_ w681]
                    seq-local: [w616 _] -> [_ w676]
                    tunnel: w605 -> [w611 _]
                    tunnel: w606 -> [w612 _]
                    tunnel: w609 -> [w625 _]
                    tunnel: w608 -> [w622 w685]
                    tunnel: w607 -> [w619 _]
                    tunnel: w604 -> [w617 _]
                    tunnel: w603 -> [_ w679]
                    tunnel: w602 -> [_ w674]
                    tunnel: [_ w680] -> w610
                    tunnel: w601 -> [w615 _]
                    tunnel: w600 -> [_ w673]
                    frame #0 {
                      n143 = Delete From Array(array=w625, length=w615, index (dim 0)=0) -> (deleted portion=w621:dbl[][][], array with subset deleted=w623:dbl[][][])  [unwired: 2 in]
                      n144 = Index Array(array=w621, index (dim 1)=0) -> (element=w614:dbl[][])  [unwired: 2 in]
                      n145 = Index Array(array=w619, index=3) -> (element=w618:T1)
                      n146 = for {
                        tunnel: w622 -> [w632] mode=indexing
                        tunnel: w614 -> [w634]
                        tunnel: w618 -> [w631]
                        tunnel: w611 -> [w630]
                        tunnel: w612 -> [w629]
                        tunnel: w617 -> [w628]
                        tunnel: [w627] -> w616
                        i -> [w626]
                        n147 = Index Array(array=w634, index (col)=w626) -> (element=w633:dbl[])  [unwired: 1 in]
                        n148 = while {
                          shift-right: [w640] -> _
                          shift-left: w633 -> [w640]
                          shift-right: [w635] -> _
                          shift-left: w632 -> [w635]
                          shift-right: [w641] -> _
                          shift-left: w631 -> [w642]
                          shift-right: [w638] -> w627
                          shift-left: w628 -> [w639]
                          shift-right: [w637] -> _
                          shift-left: w630 -> [w637]
                          shift-right: [w636] -> _
                          shift-left: w629 -> [w636]
                          stop <- w643 continue-if-true
                          n149 = call <vilib>:"H5Dget_space.vi"("obj (.)"=w635, "ref in"=w642) -> ("error out"=w649:errorcluster, "space out"=w644:T1)  [unwired: 8 in]
                          n150 = call <vilib>:"H5Sselect_simple.vi"("error in (no error)"=w649, "count"=w637, "start"=w636, "space in"=w644) -> ("error out"=w648:errorcluster, "space out"=w647:T1)  [unwired: 6 in]
                          n151 = xnode "H5Dwrite.xnode"("dataset name"=w635, "error in (no error)"=w648, "data"=w640, "file space"=w647, "ref in"=w642) -> ("error out"=w645:errorcluster)  [unwired: 2 in, 2 out]
                          n152 = call <vilib>:"H5Sclose.vi"("error in (no error)"=w645, "space in"=w644) -> ("error out"=w646:errorcluster)  [unwired: 9 in]
                          n153 = Unbundle By Name(w646) -> ("status"=w643:bool)
                          n154 = case shown="True" w643 {
                            tunnel: w642 -> [w651 _]
                            tunnel: [w651 w653] -> w641
                            tunnel: w639 -> [w650 w654]
                            tunnel: [w650 w652] -> w638
                            frame False {
                            }
                            frame True {
                              n155 = call "CloseOpenRef.vi"("Exp_params"=w654) -> ("Exp_params_out"=w652:T3, "group out"=w653:T1)  [unwired: 1 in]
                            }
                          }
                        }
                      }
                    }
                    frame #1 {
                      n156 = Unbundle By Name(w676) -> ("File Ref list"=w684:T1[])
                      n157 = call "Count2Indexes.vi"("sweep_dim"=w673, "Count"=w674) -> ("Indexes"=w675:u64[])
                      n158 = Index Array(array=w681, index (dim 1)=0) -> (element=w678:dbl[][])  [unwired: 2 in]
                      n159 = Index Array(array=w684, index=3) -> (element=w682:T1)
                      n160 = for {
                        tunnel: w685 -> [w692] mode=indexing
                        tunnel: w678 -> [w694]
                        tunnel: w682 -> [w691]
                        tunnel: w679 -> [w690]
                        tunnel: w675 -> [w689]
                        tunnel: w676 -> [w688]
                        tunnel: [w687] -> _
                        tunnel: [w687] -> w680
                        i -> [w686]
                        n161 = Index Array(array=w694, index (col)=w686) -> (element=w693:dbl[])  [unwired: 1 in]
                        n162 = while {
                          shift-right: [w700] -> _
                          shift-left: w693 -> [w700]
                          shift-right: [w696] -> _
                          shift-left: w692 -> [w696]
                          shift-right: [w701] -> _
                          shift-left: w691 -> [w702]
                          shift-right: [w698] -> w687
                          shift-left: w688 -> [w699]
                          shift-right: [w697] -> _
                          shift-left: w690 -> [w697]
                          shift-right: [w695] -> _
                          shift-left: w689 -> [w695]
                          stop <- w703 continue-if-true
                          n163 = call <vilib>:"H5Dget_space.vi"("obj (.)"=w696, "ref in"=w702) -> ("error out"=w709:errorcluster, "space out"=w704:T1)  [unwired: 8 in]
                          n164 = call <vilib>:"H5Sselect_simple.vi"("error in (no error)"=w709, "count"=w697, "start"=w695, "space in"=w704) -> ("error out"=w708:errorcluster, "space out"=w707:T1)  [unwired: 6 in]
                          n165 = xnode "H5Dwrite.xnode"("dataset name"=w696, "error in (no error)"=w708, "data"=w700, "file space"=w707, "ref in"=w702) -> ("error out"=w705:errorcluster)  [unwired: 2 in, 2 out]
                          n166 = call <vilib>:"H5Sclose.vi"("error in (no error)"=w705, "space in"=w704) -> ("error out"=w706:errorcluster)  [unwired: 9 in]
                          n167 = Unbundle By Name(w706) -> ("status"=w703:bool)
                          n168 = case shown="True" w703 {
                            tunnel: w702 -> [w711 _]
                            tunnel: [w711 w713] -> w701
                            tunnel: w699 -> [w710 w714]
                            tunnel: [w710 w712] -> w698
                            frame False {
                            }
                            frame True {
                              n169 = call "CloseOpenRef.vi"("Exp_params"=w714) -> ("Exp_params_out"=w712:T3, "group out"=w713:T1)  [unwired: 1 in]
                            }
                          }
                        }
                      }
                    }
                  }
                }
              }
            }
            frame True {
              # "buffer size smaller than the fist dim size"
              n170 = Index Array(array=w735, index (dim 1)=0) -> (element=w733:dbl[][])  [unwired: 2 in]
              n171 = stacked-sequence {
                seq-local: [w759 _] -> [_ w810]
                seq-local: [w752 _] -> [_ w817]
                tunnel: w743 -> [w751 _]
                tunnel: w744 -> [w750 _]
                tunnel: w733 -> [w762 _]
                tunnel: w747 -> [w761 _]
                tunnel: w746 -> [w758 w821]
                tunnel: w745 -> [w755 w819]
                tunnel: w748 -> [w753 _]
                tunnel: w736 -> [_ _]
                tunnel: w737 -> [_ _]
                tunnel: [_ w811] -> w749
                tunnel: w739 -> [_ w816]
                tunnel: w742 -> [_ _]
                tunnel: w741 -> [_ _]
                tunnel: w740 -> [_ w815]
                tunnel: w738 -> [_ w812]
                frame #0 {
                  n172 = Delete From Array(array=w762, length=w761, index (row)=0) -> (deleted portion=w757:dbl[][], array with subset deleted=w759:dbl[][])  [unwired: 1 in]
                  n173 = Index Array(array=w755, index=3) -> (element=w754:T1)
                  n174 = for {
                    tunnel: w758 -> [w769] mode=indexing
                    tunnel: w757 -> [w771]
                    tunnel: w754 -> [w768]
                    tunnel: w751 -> [w767]
                    tunnel: w750 -> [w766]
                    tunnel: w753 -> [w765]
                    tunnel: [w764] -> w752
                    i -> [w763]
                    n175 = Index Array(array=w771, index (col)=w763) -> (element=w770:dbl[])  [unwired: 1 in]
                    n176 = while {
                      shift-right: [w777] -> _
                      shift-left: w770 -> [w777]
                      shift-right: [w772] -> _
                      shift-left: w769 -> [w772]
                      shift-right: [w778] -> _
                      shift-left: w768 -> [w779]
                      shift-right: [w775] -> w764
                      shift-left: w765 -> [w776]
                      shift-right: [w774] -> _
                      shift-left: w767 -> [w774]
                      shift-right: [w773] -> _
                      shift-left: w766 -> [w773]
                      stop <- w780 continue-if-true
                      n177 = call <vilib>:"H5Dget_space.vi"("obj (.)"=w772, "ref in"=w779) -> ("error out"=w786:errorcluster, "space out"=w781:T1)  [unwired: 8 in]
                      n178 = call <vilib>:"H5Sselect_simple.vi"("error in (no error)"=w786, "count"=w774, "start"=w773, "space in"=w781) -> ("error out"=w785:errorcluster, "space out"=w784:T1)  [unwired: 6 in]
                      n179 = xnode "H5Dwrite.xnode"("dataset name"=w772, "error in (no error)"=w785, "data"=w777, "file space"=w784, "ref in"=w779) -> ("error out"=w782:errorcluster)  [unwired: 2 in, 2 out]
                      n180 = call <vilib>:"H5Sclose.vi"("error in (no error)"=w782, "space in"=w781) -> ("error out"=w783:errorcluster)  [unwired: 9 in]
                      n181 = Unbundle By Name(w783) -> ("status"=w780:bool)
                      n182 = case shown="True" w780 {
                        tunnel: w779 -> [w788 _]
                        tunnel: [w788 w790] -> w778
                        tunnel: w776 -> [w787 w791]
                        tunnel: [w787 w789] -> w775
                        frame False {
                        }
                        frame True {
                          n183 = call "CloseOpenRef.vi"("Exp_params"=w791) -> ("Exp_params_out"=w789:T3, "group out"=w790:T1)  [unwired: 1 in]
                        }
                      }
                    }
                  }
                }
                frame #1 {
                  n184 = Index Array(array=w815, index=0) -> (element=w813:u64)
                  n185 = Index Array(array=w819, index=3) -> (element=w818:T1)
                  n186 = while {
                    tunnel: w821 -> [w840]
                    tunnel: w818 -> [w839]
                    tunnel: w817 -> [w838]
                    tunnel: [w837] -> w811
                    shift-right: [w822] -> _
                    shift-left: w810 -> [w833]
                    tunnel: w815 -> [w830]
                    shift-right: [w831] -> _
                    shift-left: w816 -> [w829]
                    tunnel: w813 -> [w826]
                    tunnel: w812 -> [w825]
                    stop <- w832 stop-if-true
                    n187 = Array Size(array=w833) -> (size(s)=w836:i32[])
                    n188 = Index Array(array=w836, index=0) -> (element=w827:i32)
                    n189 = Greater?(x=w827, y=w826) -> (0:w834:bool)
                    n190 = case shown="True" w834 {
                      tunnel: w829 -> [w845 w860]
                      tunnel: w826 -> [_ w856]
                      tunnel: w833 -> [w847 w859]
                      tunnel: [w847 w858] -> w828
                      tunnel: [TRUE FALSE] -> w832
                      tunnel: [dbl[][] [] w849] -> w822
                      tunnel: [w845 w854] -> w831
                      tunnel: w827 -> [w842 _]
                      tunnel: w826 -> [_ w852]
                      tunnel: w825 -> [w841 w853]
                      tunnel: [w843 w850] -> w824
                      frame False {
                        n191 = Replace Array Subset(array=w841, new element=w842, index=0) -> (w843:i32[])
                      }
                      frame True {
                        n192 = Delete From Array(array=w859, length=w856, index (row)=0) -> (deleted portion=w858:dbl[][], array with subset deleted=w849:dbl[][])  [unwired: 1 in]
                        n193 = Add(x=w856, y=w860) -> (x+y=w854:u64)
                        n194 = Replace Array Subset(array=w853, new element=w852, index=0) -> (w850:i32[])
                      }
                    }
                    n195 = call "Count2Indexes.vi"("sweep_dim"=w830, "Count"=w829) -> ("Indexes"=w823:u64[])
                    n196 = for {
                      tunnel: w840 -> [w867] mode=indexing
                      tunnel: w828 -> [w869]
                      tunnel: w839 -> [w866]
                      tunnel: w838 -> [w865]
                      tunnel: [w864] -> w837
                      tunnel: w823 -> [w862]
                      tunnel: w824 -> [w863]
                      i -> [w861]
                      n197 = Index Array(array=w869, index (col)=w861) -> (element=w868:dbl[])  [unwired: 1 in]
                      n198 = while {
                        shift-right: [w875] -> _
                        shift-left: w868 -> [w875]
                        shift-right: [w872] -> _
                        shift-left: w867 -> [w872]
                        shift-right: [w876] -> _
                        shift-left: w866 -> [w877]
                        shift-right: [w873] -> w864
                        shift-left: w865 -> [w874]
                        shift-right: [w871] -> _
                        shift-left: w863 -> [w871]
                        shift-right: [w870] -> _
                        shift-left: w862 -> [w870]
                        tunnel: w863 -> [_]
                        stop <- w878 continue-if-true
                        n199 = call <vilib>:"H5Dget_space.vi"("obj (.)"=w872, "ref in"=w877) -> ("error out"=w884:errorcluster, "space out"=w879:T1)  [unwired: 8 in]
                        n200 = call <vilib>:"H5Sselect_simple.vi"("error in (no error)"=w884, "count"=w871, "start"=w870, "space in"=w879) -> ("error out"=w883:errorcluster, "space out"=w882:T1)  [unwired: 6 in]
                        n201 = xnode "H5Dwrite.xnode"("dataset name"=w872, "error in (no error)"=w883, "data"=w875, "file space"=w882, "ref in"=w877) -> ("error out"=w880:errorcluster)  [unwired: 2 in, 2 out]
                        n202 = call <vilib>:"H5Sclose.vi"("error in (no error)"=w880, "space in"=w879) -> ("error out"=w881:errorcluster)  [unwired: 9 in]
                        n203 = Unbundle By Name(w881) -> ("status"=w878:bool)
                        n204 = case shown="True" w878 {
                          tunnel: w877 -> [w886 _]
                          tunnel: [w886 w888] -> w876
                          tunnel: w874 -> [w885 w889]
                          tunnel: [w885 w887] -> w873
                          frame False {
                          }
                          frame True {
                            n205 = call "CloseOpenRef.vi"("Exp_params"=w889) -> ("Exp_params_out"=w887:T3, "group out"=w888:T1)  [unwired: 1 in]
                          }
                        }
                      }
                    }
                  }
                }
              }
            }
          }
        }
      }
    }
  }
  "count out" <- w2
  "Exp_params out" <- w1
